vi "Set MC Test Data Global.vi"(8 "error in (no error)":errorcluster, 11 "Save MC TestData":bool) -> (0 "error out":errorcluster)   [LabVIEW 2017]
uses:
  Global Variables/General Globals.vi
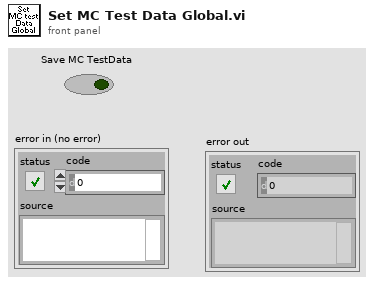
[diagram p1: front panel]
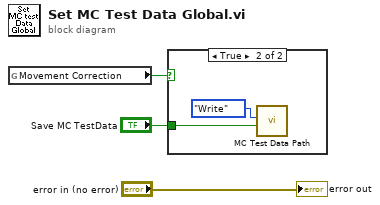
[diagram p0: block diagram]
diagram:
  n1 = global read "General Globals.vi" "Movement Correction"() -> (w3:bool)
  n2 = case shown="True" w3 {
    tunnel: "Save MC TestData" -> [_ w4]
    frame False {
    }
    frame True {
      n3 = call "MC Test Data Path.vi"("Save Test Data"=w4, "State"=enum16{"Initialise", "Write", "Read"}."Write") -> ()  [unwired: 7 in, 3 out]
    }
  }
  "error out" <- "error in (no error)"
